vi "GetEventTopicArn.vi"(8 "error in (no error)":errorcluster, 10 "Event Name":string, 11 "Refnum in":T1) -> (0 "error out":errorcluster, 3 "TopicArn":string)   [LabVIEW 2014, in "FRCts20_SNS.lvlib"]
uses:
  FRCts20_SNS.lvlib
  Backend/source/VI Source/FRCts20_Backend_Engine.lvlib
  <vilib>/addons/database/Connection.llb/Conn ObjectReference.ctl
  <vilib>/addons/database/NI_Database_API.lvlib
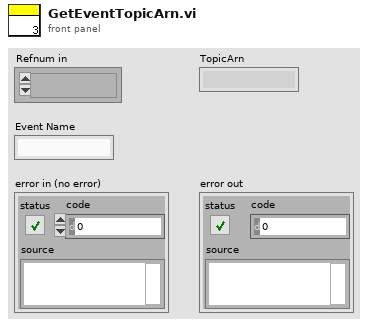
[diagram p1: front panel]
types:
  T1 = typedef "NI_Database_API.lvlib/Conn ObjectReference.ctl" = refnum<k1>
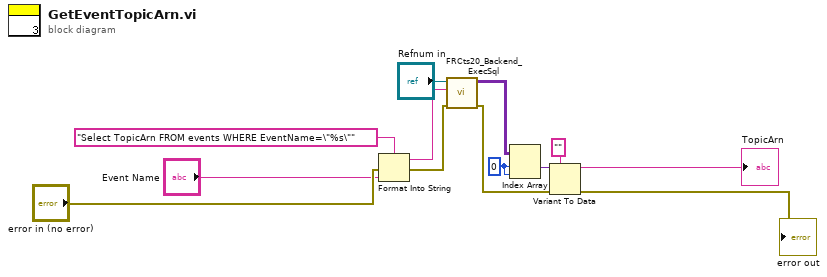
[diagram p0: block diagram]
diagram:
  w3 = 0 ("index (row)")
  n1 = Format Into String(format string="Select TopicArn FROM events WHERE EventName=\"%s\"" ("TopicArn"), error in="error in (no error)", "Event Name") -> (resulting string=w7:string, error out=w11:errorcluster)  [unwired: 1 in]
  n2 = call "FRCts20_Backend_ExecSql.vi"("error in (no error)"=w11, "format string"=w7, "Refnum in"="Refnum in") -> ("error out"=w12:errorcluster, "recordset data"=w4:variant[][])  [unwired: 6 in, 1 out]
  n3 = Index Array(array=w4, index (row)=w3, index (col)=w3) -> (element=w2:variant)
  n4 = Variant To Data(error in=w12, type="" ("TopicArn"), Variant=w2) -> (data=→"TopicArn":string, error out=→"error out":errorcluster)
